vi "Initialize & Run FPGA.vi"(8 "error in (no error)":errorcluster, 11 "Refnum in":T1) -> (0 "error out":errorcluster, 2 "FPGA VI Execution Mode":T2, 3 "Refnum out":T1)   [LabVIEW 2014]
uses:
  <vilib>/FPGA/interface/niFpgaViExecutionMode.ctl
  Type Definitions/FPGA Reference.ctl
  <vilib>/rvi/interface/common/dynamic/niFpgaDynamicGetExecutionMode.vi
  <vilib>/FPGAPlugInAG/Dynamic/niLvFpga_Reset_Dynamic.vi
  <vilib>/rvi/interface/common/niFpgaWaitOnOcc.vi
  <vilib>/Utility/error.llb/Error Cluster From Error Code.vi
  <vilib>/FPGAPlugInAG/Dynamic/niLvFpga_Run_Dynamic.vi
  <vilib>/rvi/interface/nirviMethod/nirviMethod.xnode
  <vilib>/FPGAPlugInAG/Dynamic/niLvFpga_ConfigureFifo_Dynamic.vi
  <vilib>/rvi/errors/niLvFpgaMergeErrorWithErrorCode.vi
  <vilib>/FPGAPlugInAG/Dynamic/niLvFpga_StartFifo_Dynamic.vi
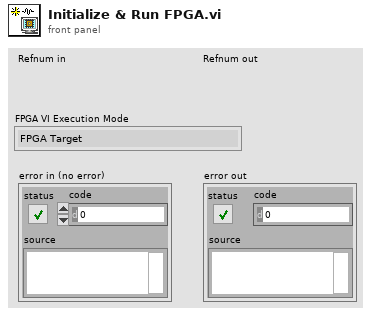
[diagram p1: front panel]
types:
  T1 = typedef "FPGA Reference.ctl" = refnum<k20>
  T2 = typedef "niFpgaViExecutionMode.ctl" = enum16{"FPGA Target", "Simulation (Simulated I/O)", "Simulation (Real I/O)", "Third-Party Simulation"}
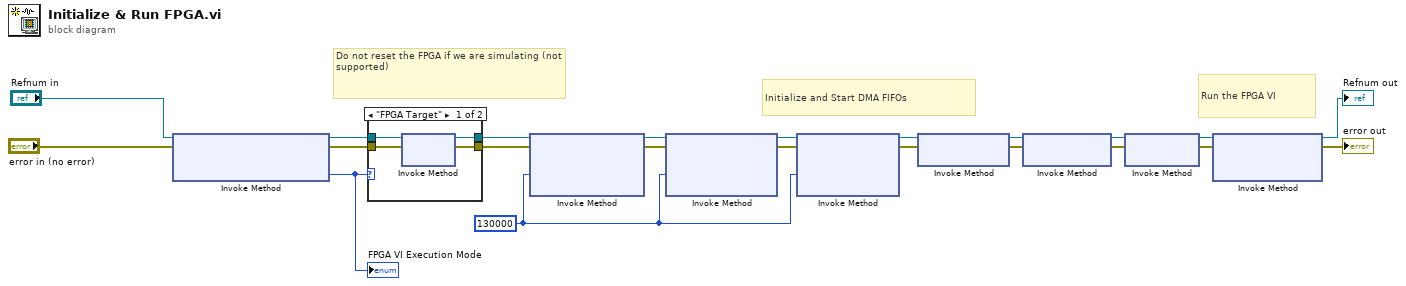
[diagram p0: block diagram]
diagram:
  w1 = u32 130000
  # "Run the FPGA VI"
  # "Initialize and Start DMA FIFOs"
  # "Do not reset the FPGA if we are simulating (not supported)"
  n1 = xnode "Invoke Method"("FPGA VI Reference In"="Refnum in", "error in"="error in (no error)") -> ("FPGA VI Reference Out"=w18:T1, "error out"=w17:errorcluster, "FPGA VI Execution Mode"=w2:T2)
  "FPGA VI Execution Mode" <- w2
  n2 = case shown="\"FPGA Target\"" w2 {
    tunnel: [w26 w28] -> w20
    tunnel: w17 -> [w25 w28]
    tunnel: w18 -> [w24 w27]
    tunnel: [w23 w27] -> w19
    frame "FPGA Target" {
      n3 = xnode "Invoke Method"("FPGA VI Reference In"=w24, "error in"=w25) -> ("FPGA VI Reference Out"=w23:T1, "error out"=w26:errorcluster)
    }
    frame "Simulation (Simulated I/O)", Default {
    }
  }
  n4 = xnode "Invoke Method"("FPGA VI Reference In"=w19, "error in"=w20, "Requested Depth"=w1) -> ("FPGA VI Reference Out"=w7:T1, "error out"=w5:errorcluster)  [unwired: 1 out]
  n5 = xnode "Invoke Method"("FPGA VI Reference In"=w7, "error in"=w5, "Requested Depth"=w1) -> ("FPGA VI Reference Out"=w6:T1, "error out"=w4:errorcluster)  [unwired: 1 out]
  n6 = xnode "Invoke Method"("FPGA VI Reference In"=w6, "error in"=w4, "Requested Depth"=w1) -> ("FPGA VI Reference Out"=w21:T1, "error out"=w22:errorcluster)  [unwired: 1 out]
  n7 = xnode "Invoke Method"("FPGA VI Reference In"=w21, "error in"=w22) -> ("FPGA VI Reference Out"=w14:T1, "error out"=w12:errorcluster)
  n8 = xnode "Invoke Method"("FPGA VI Reference In"=w14, "error in"=w12) -> ("FPGA VI Reference Out"=w15:T1, "error out"=w13:errorcluster)
  n9 = xnode "Invoke Method"("FPGA VI Reference In"=w15, "error in"=w13) -> ("FPGA VI Reference Out"=w11:T1, "error out"=w10:errorcluster)
  n10 = xnode "Invoke Method"("FPGA VI Reference In"=w11, "error in"=w10) -> ("FPGA VI Reference Out"=→"Refnum out":T1, "error out"=→"error out":errorcluster)  [unwired: 1 in]
